vi "Assert Array Contains.vi"(4 "Execution time (s)":dbl=-1.0, 5 "Assert Only? (F)":bool, 6 "error code (1)":i32=1, 7 "Label (\"\")":string, 8 "error in (no error)":errorcluster, 9 "Register with caller test (F)":bool, 10 "Element":variant, 11 "Array":variant) -> (0 "error out":errorcluster, 2 "Properties.Assert":refnum<class "Properties.Assert.lvclass">)   [LabVIEW 2013, in "Caraya.lvlib" / "Assert.lvclass"]
doc: "Asserts that an array contains a specific element."
uses:
  Assert.lvclass
  Properties.Assert/Properties.Assert.lvclass
  Properties/Properties.lvclass
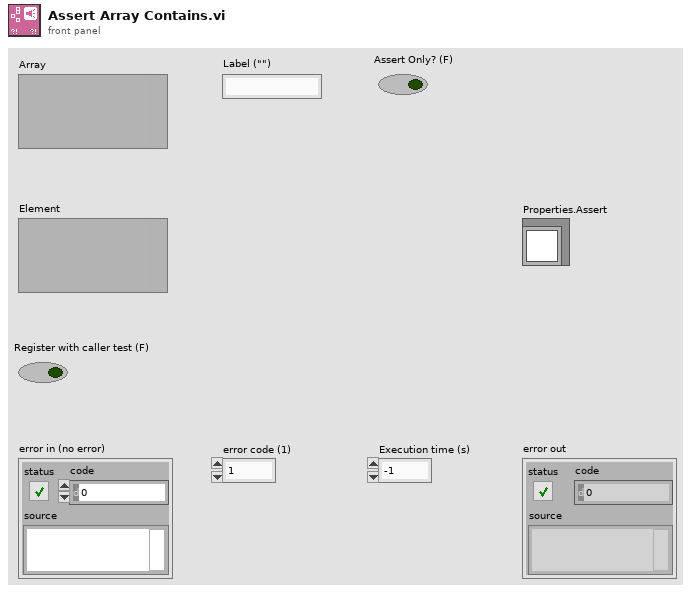
[diagram p1: front panel]
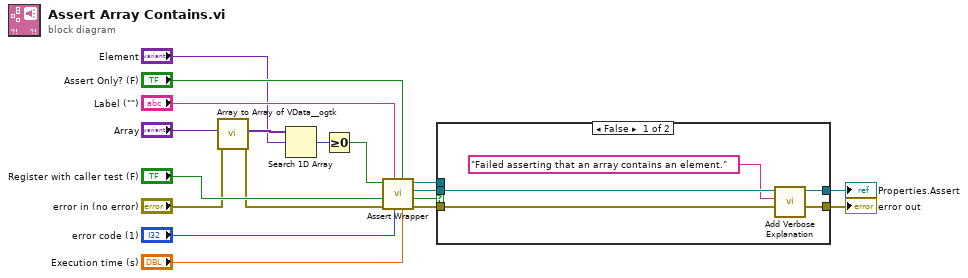
[diagram p0: block diagram]
diagram:
  n1 = call <userlib>:"Array to Array of VData__ogtk.vi"("error in (no error)"="error in (no error)", "MultiD Array"="Array") -> ("error out"=w1:errorcluster, "1D Array of Variants"=w7:variant[])  [unwired: 8 in]
  n2 = Search 1D Array(1D array=w7, element="Element") -> (index of element=w6:i32)  [unwired: 1 in]
  n3 = Greater Or Equal To 0?(x=w6) -> (x >= 0?=w5:bool)
  n4 = call "Assert Wrapper.vi"("Execution time (s)"="Execution time (s)", "Assert Only? (F)"="Assert Only? (F)", "error code (1)"="error code (1)", "Label"="Label (\"\")", "error in (no error)"=w1, "Register with caller test (F)"="Register with caller test (F)", "Assert?"=w5) -> ("error out"=w9:errorcluster, "Verbose"=w13:bool, "Properties.Assert"=w11:refnum<class "Properties.Assert.lvclass">, "Assert out"=w12:refnum<class "Assert.lvclass">)  [unwired: 1 in]
  n5 = case shown="False" w13 {
    tunnel: w12 -> [_ _]
    tunnel: w11 -> [w21 w25]
    tunnel: [w22 w24] -> w10
    tunnel: w9 -> [w23 w24]
    tunnel: [w20 w25] -> w8
    frame False {
      n6 = call "Add Verbose Explanation.vi"("error in (no error)"=w23, "Verbose Explanation"="Failed asserting that an array contains an element.", "Properties"=w21) -> ("error out"=w22:errorcluster, "Properties"=w20:refnum<class "Properties.Assert.lvclass">)  [unwired: 7 in]
    }
    frame True {
    }
  }
  "error out" <- w10
  "Properties.Assert" <- w8
